vi "Read Key (I32).vi"(7 "Section Name":string, 8 "error in (no error)":errorcluster, 9 "Default":i32, 10 "Key Name":string, 11 "Config in":T1) -> (0 "error out":errorcluster, 1 "Value":i32, 2 "Key Found?":bool, 3 "Config out":T1)   [LabVIEW 2022 SP3, in "LabVIEW-Config.lvlib"]
uses:
  LabVIEW-Config.lvlib
  Config.ctl
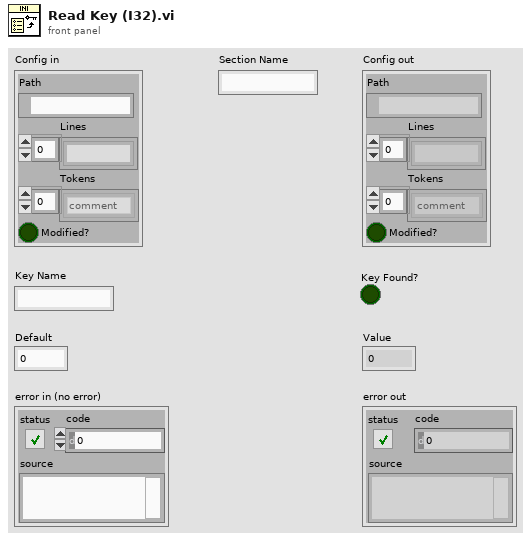
[diagram p1: front panel]
types:
  T1 = typedef "LabVIEW-Config.lvlib/Config.ctl" = cluster{"Path":path, "Lines":string[], "Tokens":enum8{"comment", "section", "key"}[], "Modified?":bool}
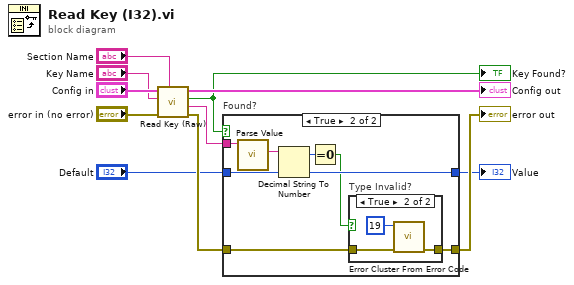
[diagram p0: block diagram]
diagram:
  n1 = call "Read Key (Raw).vi"("Section Name"="Section Name", "error in (no error)"="error in (no error)", "Key Name"="Key Name", "Config in"="Config in") -> ("error out"=w4:errorcluster, "Content"=w6:string, "Key Found?"=w3:bool, "Config out"=→"Config out":T1)  [unwired: 4 in]
  "Key Found?" <- w3
  n2 = case "Found?" shown="True" w3 {
    tunnel: w6 -> [_ w21]
    tunnel: [w13 w15] -> w1
    tunnel: "Default" -> [w13 w16]
    tunnel: [w12 w20] -> w5
    tunnel: w4 -> [w12 w19]
    frame False {
    }
    frame True {
      n3 = call "Parse Value.vi"("Value"=w21) -> ("Value (Comment Removed)"=w17:string)  [unwired: 9 in, 1 out]
      n4 = Decimal String To Number(string=w17, default (0L)=w16) -> (offset past number=w18:i32, number=w15:i32)  [unwired: 1 out]
      n5 = Equal To 0?(x=w18) -> (x = 0?=w14:bool)
      n6 = case "Type Invalid?" shown="True" w14 {
        tunnel: w19 -> [w22 w24]
        tunnel: [w22 w23] -> w20
        frame False {
        }
        frame True {
          n7 = call <vilib>:"Error Cluster From Error Code.vi"("error in (no error)"=w24, "error code (0)"=19 ("Type invalid")) -> ("error out"=w23:errorcluster)  [unwired: 7 in]
        }
      }
    }
  }
  "error out" <- w5
  "Value" <- w1
